vi "Fixed VI.vi"() -> ()   [LabVIEW 2010]
panel:
  out "Running Result":dbl
  in  "X":dbl
  in  "Calculate":bool
  in  "Action":T1(ring)
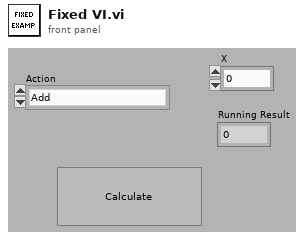
[diagram p1: front panel]
types:
  T1 = enum16{"Add", "Subtract", "Multiply", "Divide", "Set"}
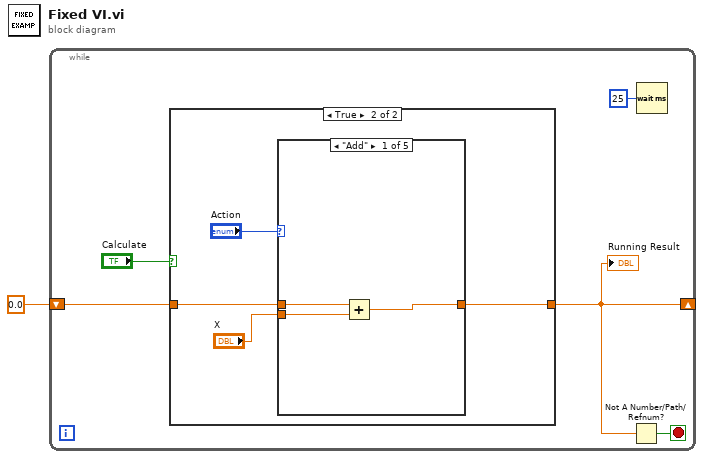
[diagram p0: block diagram]
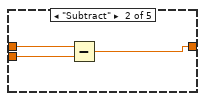
[diagram p3: hidden frame]
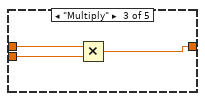
[diagram p4: hidden frame]
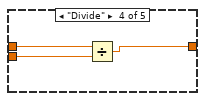
[diagram p5: hidden frame]
diagram:
  n1 = while {
    shift-right: [w4] -> _
    shift-left: 0.0 -> [w6]
    stop <- w3 stop-if-true
    n2 = case shown="True" "Calculate" {
      tunnel: w6 -> [w7 w10]
      tunnel: [w7 w9] -> w4
      frame False {
      }
      frame True {
        n3 = case shown="\"Add\"" "Action" {
          tunnel: w10 -> [w13 w17 w20 w23 _]
          tunnel: [w14 w15 w18 w21 w24] -> w9
          tunnel: "X" -> [w12 w16 w19 w22 w24]
          frame "Add" {
            n4 = Add(x=w13, y=w12) -> (x+y=w14:dbl)
          }
          frame "Subtract" {
            n5 = Subtract(x=w17, y=w16) -> (x-y=w15:dbl)
          }
          frame "Multiply" {
            n6 = Multiply(x=w20, y=w19) -> (x*y=w18:dbl)
          }
          frame "Divide" {
            n7 = Divide(x=w23, y=w22) -> (x/y=w21:dbl)
          }
          frame "Set", Default {
          }
        }
      }
    }
    "Running Result" <- w4
    n8 = Not A Number/Path/Refnum?(number/path/refnum=w4) -> (NaN/Path/Refnum?=w3:bool)
    n9 = Wait (ms)(milliseconds to wait=u32 25) -> ()  [unwired: 1 out]
  }
